vi "Lookup Running Measurement Queue.vi"(8 "error in (no error)":errorcluster, 10 "Measurement Name.Harware()":string, 11 "Controller in":refnum<class "Controller.lvclass">) -> (0 "error out":errorcluster, 1 "Measurement Queue":refnum<class "Message Enqueuer.lvclass">, 2 "Found?":bool, 3 "Controller out":refnum<class "Controller.lvclass">)   [LabVIEW 2015, in "Controller Actor.lvlib" / "Controller.lvclass"]
uses:
  Controller.lvclass
  <vilib>/ActorFramework/Message Enqueuer/Message Enqueuer.lvclass
panel:
  in  "Self Enqueuer":refnum<class "Message Enqueuer.lvclass">
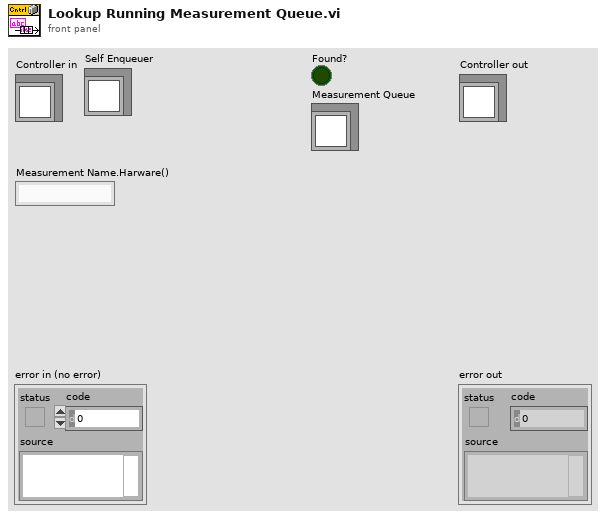
[diagram p1: front panel]
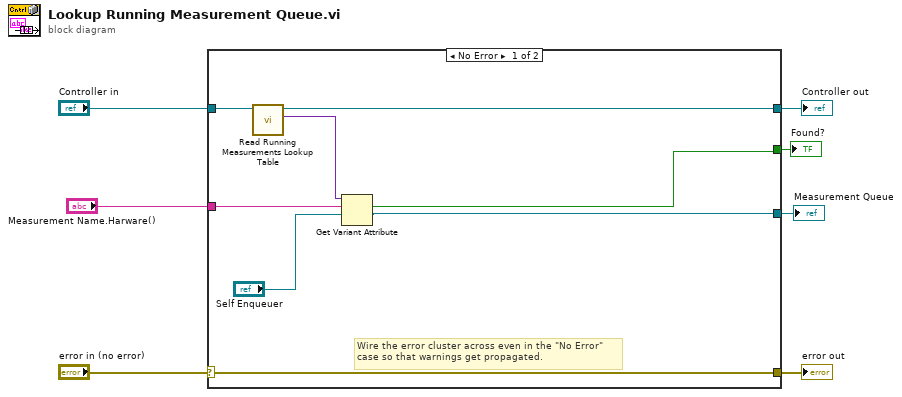
[diagram p0: block diagram]
diagram:
  n1 = case shown="No Error" "error in (no error)" {
    selector: "error in (no error)" -> [w15 w17]
    tunnel: [w15 w17] -> w6
    tunnel: [w11 w16] -> w4
    tunnel: "Controller in" -> [w12 w16]
    tunnel: "Measurement Name.Harware()" -> [w13 _]
    tunnel: [w10 _] -> w1
    tunnel: [w9 _] -> w2
    frame No Error {
      # "Wire the error cluster across even in the \"No Error\"\ncase so that warnings get propagated."
      n2 = call "Read Running Measurements Lookup Table.vi"("Controller in"=w12) -> ("Running Measurements Lookup Table"=w14:variant, "Controller out"=w11:refnum<class "Controller.lvclass">)  [unwired: 8 in, 1 out]
      n3 = Get Variant Attribute(Variant=w14, name=w13, default value (empty Variant)="Self Enqueuer") -> (found=w9:bool, value=w10:refnum<class "Message Enqueuer.lvclass">)  [unwired: 1 in, 2 out]
    }
    frame Error {
    }
  }
  "error out" <- w6
  "Controller out" <- w4
  "Found?" <- w2
  "Measurement Queue" <- w1
